vi "02TRM800.vi"() -> ()   [LabVIEW 2015]
uses:
  02TRM800_States.ctl
  <vilib>/Instr/_visa.llb/VISA Configure Serial Port (Serial Instr).vi
panel:
  in  "Tab Control":enum32{"Page 1", "Page 2"}(tab)
  out "String":string
  in  "mph":dbl min=0.0 max=16.0 step=0.1 format="%.1g"
  in  "inc":dbl min=0.0 max=15.0 step=0.5 format="%.1g"
  out "ReplyCounter":u32
  out "StringReply":string
  out "NextCommand":string
  in  "stop":bool
  in  "Serial Port":refnum<visa-resource-name>
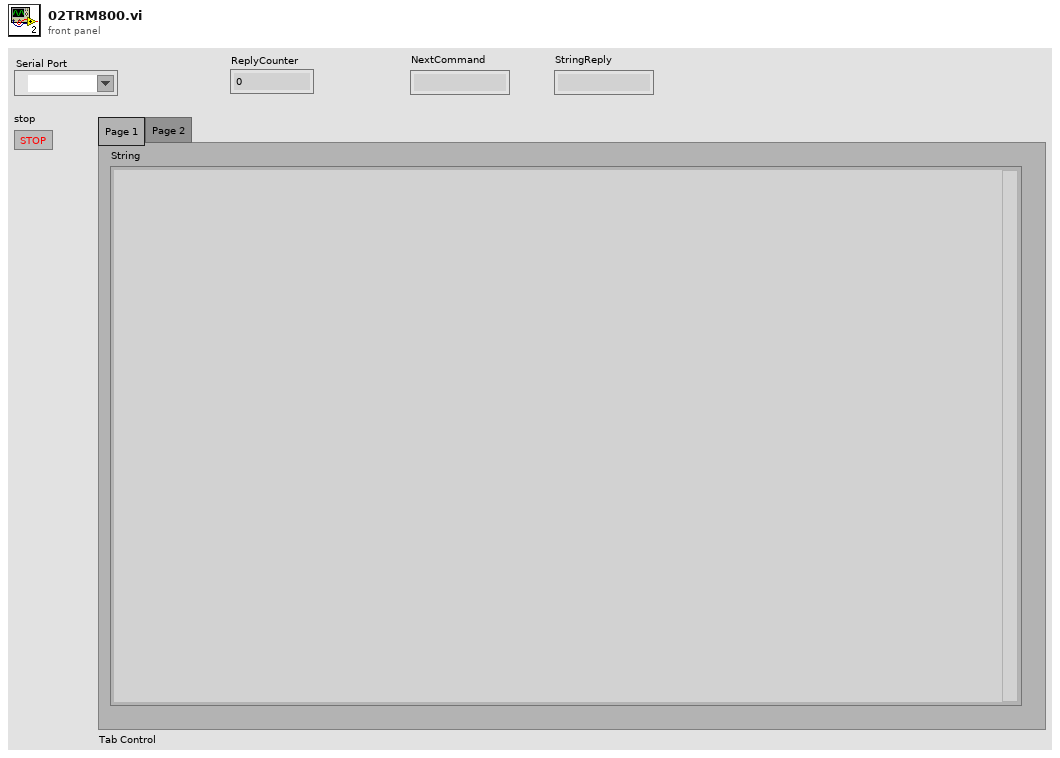
[diagram p1: front panel]
types:
  T1 = typedef "02TRM800_States.ctl" = enum16{"Initialize", "Close", "Query", "GetNext", "AnalyzeRead", "GetErrRSET", "SetMPH", "SetInc"}
  T2 = enum16{"Initialize", "Get", "SetInitCommands", "SetMPH", "SetInc"}
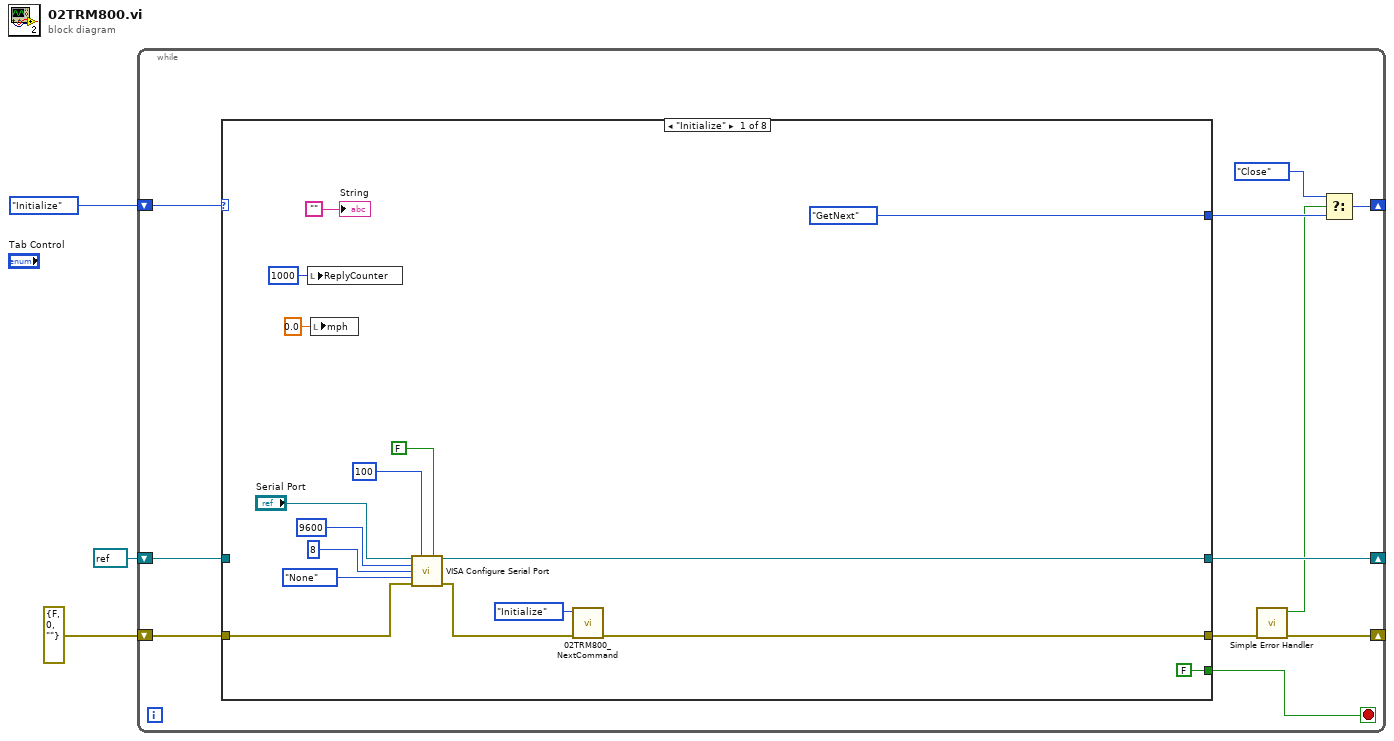
[diagram p0: block diagram]
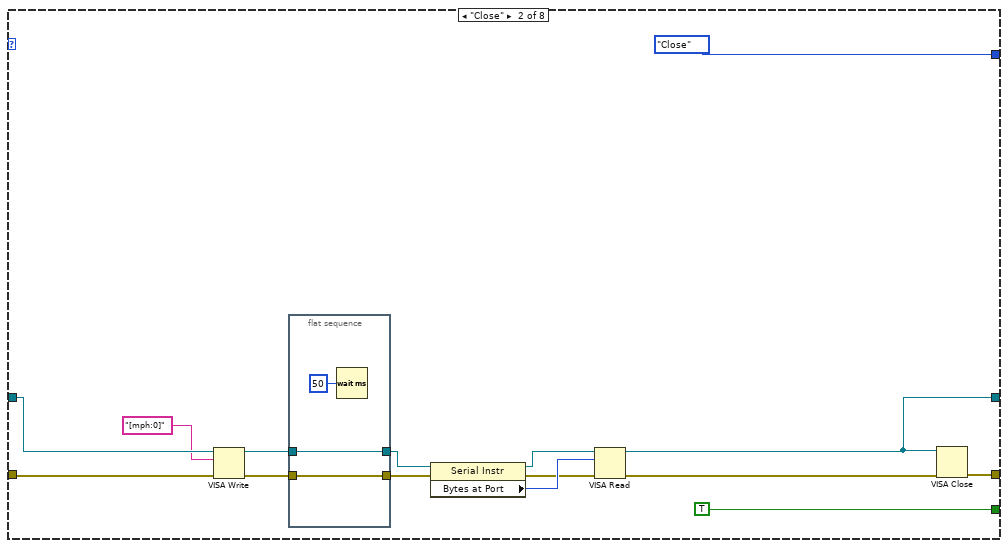
[diagram p2: hidden frame]
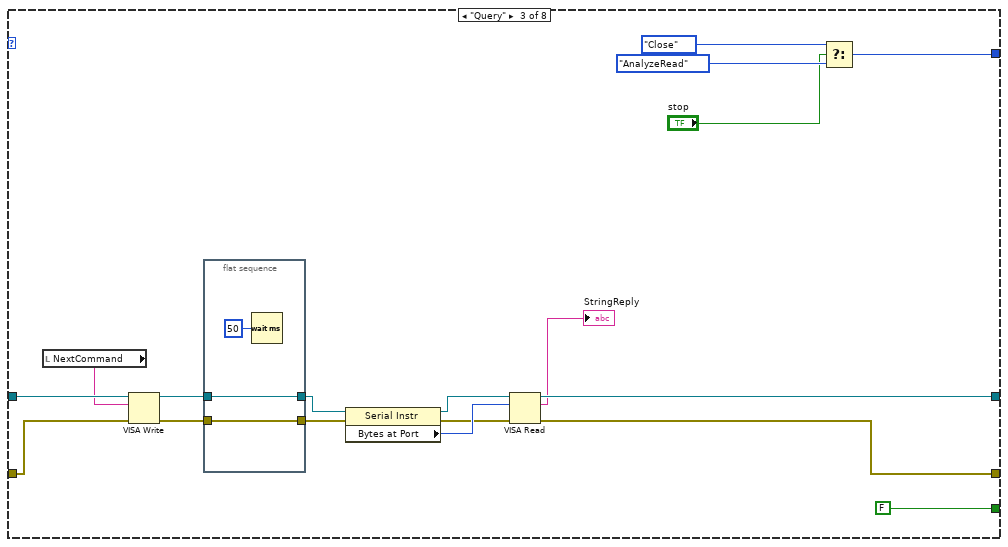
[diagram p3: hidden frame]
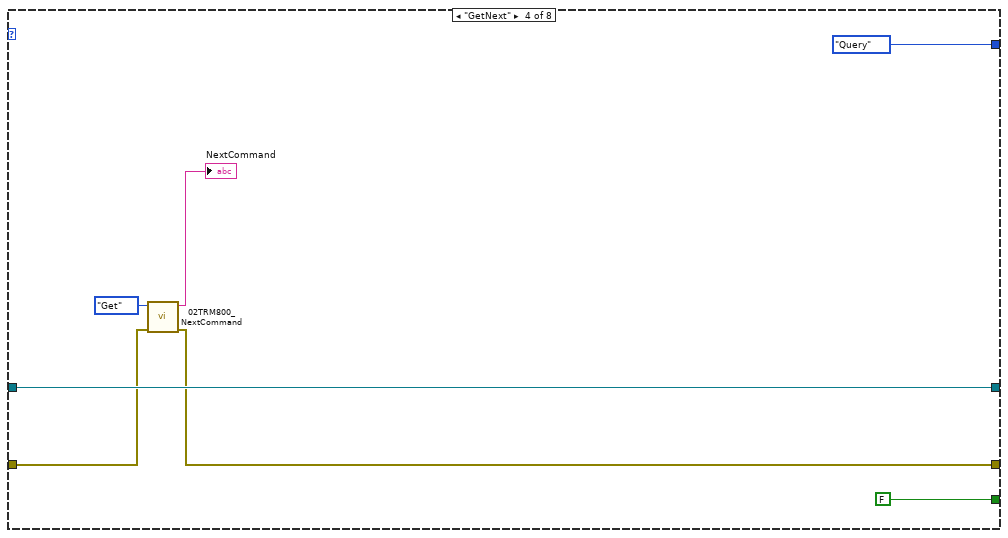
[diagram p4: hidden frame]
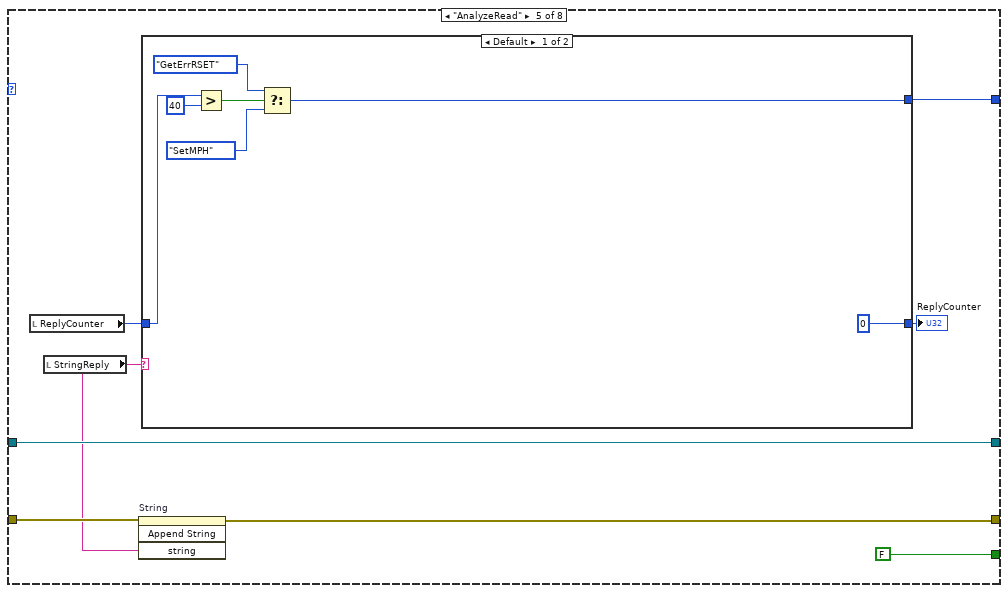
[diagram p5: hidden frame]
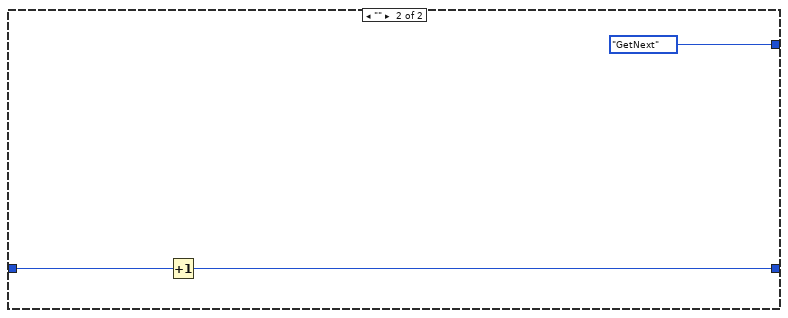
[diagram p6: hidden frame]
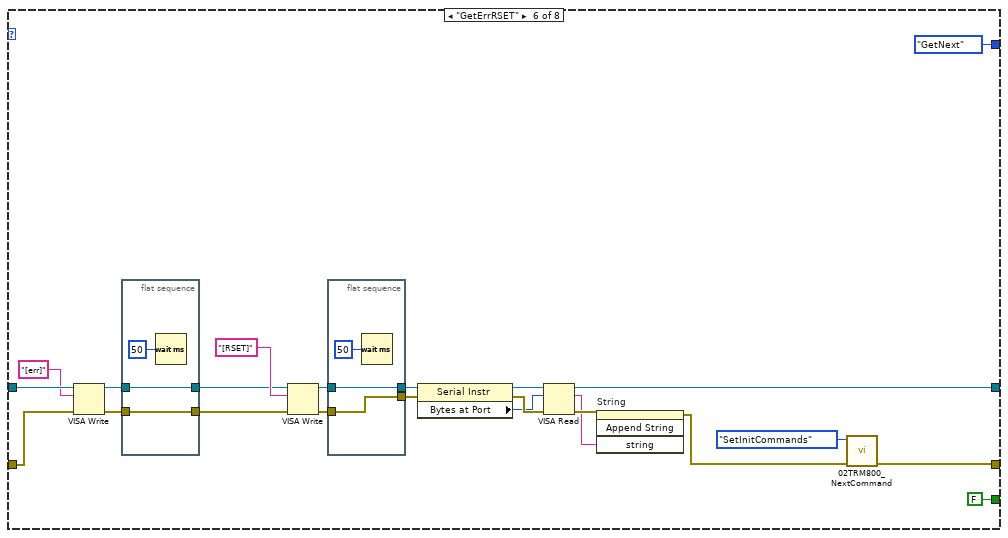
[diagram p7: hidden frame]
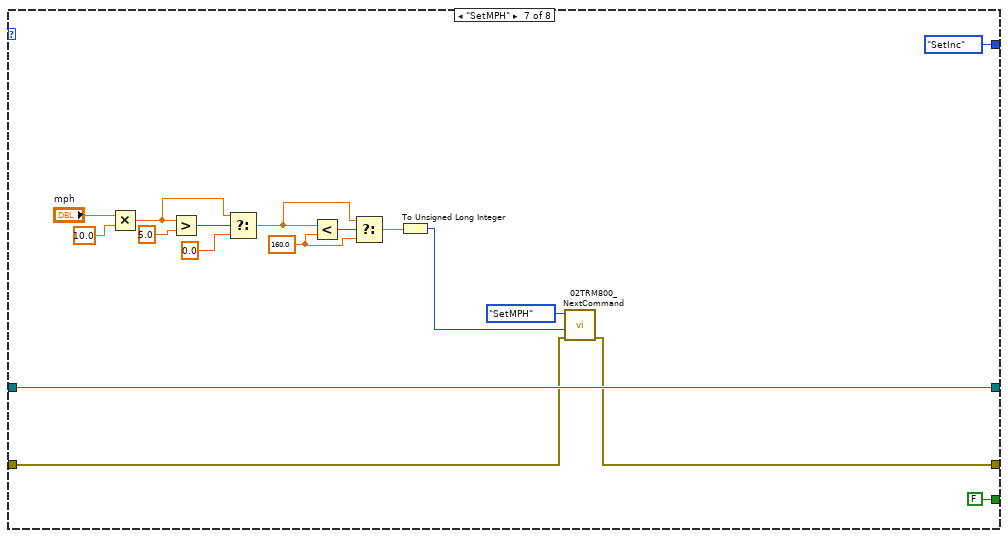
[diagram p8: hidden frame]
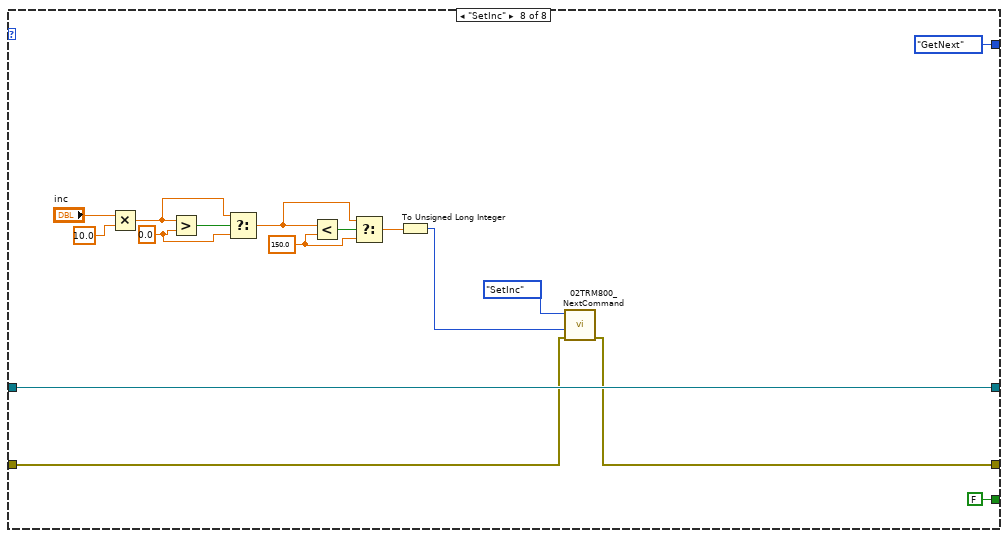
[diagram p9: hidden frame]
diagram:
  n1 = while {
    shift-right: [w10] -> _
    shift-left: errorcluster {"status"=FALSE, "code"=0, "source"=""} ("error constant") -> [w14]
    shift-right: [w6] -> _
    shift-left: 02TRM800_States."Initialize" -> [w13]
    shift-right: [w9] -> _
    shift-left: refnum<visa-resource-name> refnum ("VISA resource name out") -> [w8]
    stop <- w11 stop-if-true
    n2 = case shown="\"Initialize\"" w13 {
      tunnel: w14 -> [w25 w33 w65 w73 w84 w116 w138 w154]
      tunnel: [w19 w44 w49 w72 w82 w98 w137 w153] -> w12
      tunnel: [FALSE TRUE FALSE FALSE FALSE FALSE FALSE FALSE] -> w11
      tunnel: [02TRM800_States."GetNext" 02TRM800_States."Close" w61 02TRM800_States."Query" w77 02TRM800_States."GetNext" 02TRM800_States."SetInc" 02TRM800_States."GetNext"] -> w5
      tunnel: [w22 w34 w52 w75 w83 w100 w139 w155] -> w9
      tunnel: w8 -> [_ w35 w66 w75 w83 w117 w139 w155]
      frame "Initialize" {
        n3 = local write "ReplyCounter"(u32 1000 ("ReplyCounter")) -> ()
        n4 = local write "mph"(0.0 ("mph")) -> ()
        n5 = call-poly "VISA Configure Serial Port"("VISA resource name"="Serial Port", "timeout (10sec)"=u32 100, "Enable Termination\nChar (T)"=FALSE ("Enable Termination\nChar (T)"), "baud rate (9600)"=u32 9600, "data bits (8)"=u16 8, "parity (0:none)"=enum16{"None", "Odd", "Even", "Mark", "Space"}."None", "error in (no error)"=w25) -> ("VISA resource name out"=w22:refnum<visa-resource-name>, "error out"=w18:errorcluster)  [unwired: 7 in]
        n6 = call "02TRM800_NextCommand.vi"("error in (no error)"=w18, "Command"=enum16{"Initialize", "Get"}."Initialize") -> ("error out"=w19:errorcluster)  [unwired: 8 in, 1 out]
        "String" <- ""
      }
      frame "Close" {
        n7 = VISA Write(VISA resource name=w35, write buffer="[mph:0]", error in (no error)=w33) -> (VISA resource name out=w42:refnum<visa-resource-name>, error out=w41:errorcluster)  [unwired: 1 out]
        n8 = flat-sequence {
          tunnel: w42 -> [w47]
          tunnel: w41 -> [w46]
          tunnel: [w47] -> w40
          tunnel: [w46] -> w39
          frame #0 {
            n9 = Wait (ms)(milliseconds to wait=u32 50) -> ()  [unwired: 1 out]
          }
        }
        n10 = property class="Serial Instr"(reference=w40, error in=w39) -> (reference out=w37:refnum<visa-resource-name>, error out=w36:errorcluster, "Bytes at Port"=w38:u32)
        n11 = VISA Read(VISA resource name=w37, byte count=w38, error in (no error)=w36) -> (VISA resource name out=w34:refnum<visa-resource-name>, error out=w32:errorcluster)  [unwired: 2 out]
        n12 = VISA Close(VISA resource name=w34, error in (no error)=w32) -> (error out=w44:errorcluster)
      }
      frame "Query" {
        n13 = local read "NextCommand"() -> (w51:string)
        n14 = VISA Write(VISA resource name=w66, write buffer=w51, error in (no error)=w65) -> (VISA resource name out=w64:refnum<visa-resource-name>, error out=w63:errorcluster)  [unwired: 1 out]
        n15 = flat-sequence {
          tunnel: w64 -> [w68]
          tunnel: w63 -> [w67]
          tunnel: [w68] -> w59
          tunnel: [w67] -> w58
          frame #0 {
            n16 = Wait (ms)(milliseconds to wait=u32 50) -> ()  [unwired: 1 out]
          }
        }
        n17 = property class="Serial Instr"(reference=w59, error in=w58) -> (reference out=w55:refnum<visa-resource-name>, error out=w53:errorcluster, "Bytes at Port"=w56:u32)
        n18 = VISA Read(VISA resource name=w55, byte count=w56, error in (no error)=w53) -> (VISA resource name out=w52:refnum<visa-resource-name>, read buffer=→"StringReply":string, error out=w49:errorcluster)  [unwired: 1 out]
        n19 = Select(t=02TRM800_States."Close", s="stop", f=02TRM800_States."AnalyzeRead") -> (s? t:f=w61:T1)
      }
      frame "GetNext" {
        n20 = call "02TRM800_NextCommand.vi"("error in (no error)"=w73, "Command"=enum16{"Initialize", "Get", "SetInitCommands"}."Get") -> ("error out"=w72:errorcluster, "String"=→"NextCommand":string)  [unwired: 8 in]
      }
      frame "AnalyzeRead" {
        n21 = local read "ReplyCounter"() -> (w79:u32)
        n22 = local read "StringReply"() -> (w80:string)
        n23 = invoke on="String" class="Str" method="Append String"(error in=w84, "string"=w80) -> (error out=w82:errorcluster)  [unwired: 2 in, 3 out]
        n24 = case shown="Default" w80 {
          tunnel: w79 -> [w90 w94]
          tunnel: [u32 0 w93] -> w78
          tunnel: [w85 02TRM800_States."GetNext"] -> w77
          frame Default {
            n25 = Greater?(x=w90, y=u32 40) -> (0:w88:bool)
            n26 = Select(t=02TRM800_States."GetErrRSET", s=w88, f=02TRM800_States."SetMPH") -> (s? t:f=w85:T1)
          }
          frame "" {
            n27 = Increment(x=w94) -> (x+1=w93:u32)
          }
        }
        "ReplyCounter" <- w78
      }
      frame "GetErrRSET" {
        n28 = VISA Write(VISA resource name=w117, write buffer="[err]", error in (no error)=w116) -> (VISA resource name out=w113:refnum<visa-resource-name>, error out=w114:errorcluster)  [unwired: 1 out]
        n29 = flat-sequence {
          tunnel: w114 -> [w122]
          tunnel: w113 -> [w123]
          tunnel: [w123] -> w103
          tunnel: [w122] -> w102
          frame #0 {
            n30 = Wait (ms)(milliseconds to wait=u32 50) -> ()  [unwired: 1 out]
          }
        }
        n31 = VISA Write(VISA resource name=w103, write buffer="[RSET]", error in (no error)=w102) -> (VISA resource name out=w106:refnum<visa-resource-name>, error out=w105:errorcluster)  [unwired: 1 out]
        n32 = flat-sequence {
          tunnel: w105 -> [w119]
          tunnel: w106 -> [w120]
          tunnel: [w120] -> w110
          tunnel: [w119] -> w111
          frame #0 {
            n33 = Wait (ms)(milliseconds to wait=u32 50) -> ()  [unwired: 1 out]
          }
        }
        n34 = property class="Serial Instr"(reference=w110, error in=w111) -> (reference out=w108:refnum<visa-resource-name>, error out=w109:errorcluster, "Bytes at Port"=w107:u32)
        n35 = VISA Read(VISA resource name=w108, byte count=w107, error in (no error)=w109) -> (VISA resource name out=w100:refnum<visa-resource-name>, read buffer=w95:string, error out=w104:errorcluster)  [unwired: 1 out]
        n36 = invoke on="String" class="Str" method="Append String"(error in=w104, "string"=w95) -> (error out=w99:errorcluster)  [unwired: 2 in, 3 out]
        n37 = call "02TRM800_NextCommand.vi"("error in (no error)"=w99, "Command"=enum16{"Initialize", "Get", "SetInitCommands"}."SetInitCommands") -> ("error out"=w98:errorcluster)  [unwired: 8 in, 1 out]
      }
      frame "SetMPH" {
        w127 = 160.0 ("y")
        n38 = Multiply(x="mph", y=10.0) -> (x*y=w131:dbl)
        n39 = Greater?(x=w131, y=5.0) -> (0:w132:bool)
        n40 = Select(t=w131, s=w132, f=0.0) -> (s? t:f=w128:dbl)
        n41 = Less?(x=w128, y=w127) -> (x < y?=w129:bool)
        n42 = Select(t=w128, s=w129, f=w127) -> (s? t:f=w126:dbl)
        n43 = To Unsigned Long Integer(number=w126) -> (unsigned 32bit integer=w125:u32)
        n44 = call "02TRM800_NextCommand.vi"("error in (no error)"=w138, "Numeric"=w125, "Command"=T2."SetMPH") -> ("error out"=w137:errorcluster)  [unwired: 7 in, 1 out]
      }
      frame "SetInc" {
        w145 = 150.0 ("y")
        w141 = 0.0 ("y")
        n45 = Multiply(x="inc", y=10.0) -> (x*y=w148:dbl)
        n46 = Greater?(x=w148, y=w141) -> (0:w149:bool)
        n47 = Select(t=w148, s=w149, f=w141) -> (s? t:f=w146:dbl)
        n48 = Less?(x=w146, y=w145) -> (x < y?=w147:bool)
        n49 = Select(t=w146, s=w147, f=w145) -> (s? t:f=w144:dbl)
        n50 = To Unsigned Long Integer(number=w144) -> (unsigned 32bit integer=w143:u32)
        n51 = call "02TRM800_NextCommand.vi"("error in (no error)"=w154, "Numeric"=w143, "Command"=T2."SetInc") -> ("error out"=w153:errorcluster)  [unwired: 7 in, 1 out]
      }
    }
    n52 = call <vilib>:"Simple Error Handler.vi"("error in (no error)"=w12) -> ("error?"=w4:bool, "error out"=w10:errorcluster)  [unwired: 4 in, 3 out]
    n53 = Select(t=02TRM800_States."Close", s=w4, f=w5) -> (s? t:f=w6:T1)
  }
